vi "Write Value.vi"(8 "Error In":errorcluster, 10 "Value":dbl, 11 "Add Value without TS Msg":refnum<class "Add Value without TS Msg.lvclass">) -> (0 "Error Out":errorcluster, 3 "Add Value without TS Msg":refnum<class "Add Value without TS Msg.lvclass">)   [LabVIEW 2018, in "BNT_XtGraph.lvlib" / "Add Value without TS Msg.lvclass"]
uses:
  Add Value without TS Msg.lvclass
  Add Value without TS Msg.lvclass/Add Value without TS Msg.ctl
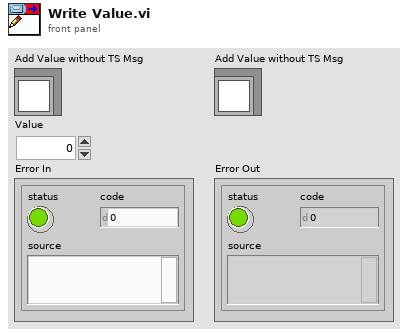
[diagram p1: front panel]
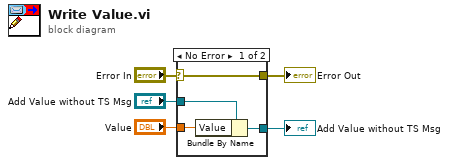
[diagram p0: block diagram]
diagram:
  n1 = case shown="No Error" "Error In" {
    selector: "Error In" -> [w9 w10]
    tunnel: [w9 w10] -> w5
    tunnel: [w7 w11] -> w3
    tunnel: "Add Value without TS Msg" -> [w8 w11]
    tunnel: "Value" -> [w6 _]
    frame No Error {
      n2 = Bundle By Name(cluster=w8, "Value"=w6) -> (w7:refnum<class "Add Value without TS Msg.lvclass">)
    }
    frame Error {
    }
  }
  "Add Value without TS Msg" <- w3
  "Error Out" <- w5
